vi "H5Diterate_cbhelper.vi"(5 "VI Refnum":refnum<vi>, 6 "error in (no error)":errorcluster, 7 "point":u64[](array[numeric]), 8 "User data in":variant, 9 "Data array in":variant) -> (0 "error out":errorcluster, 1 "Stop":i32(ring) items=["Error"=-1, "Continue"=0, "Stop"=1], 2 "User data out":variant, 3 "Data array out":variant)   [LabVIEW 2017]
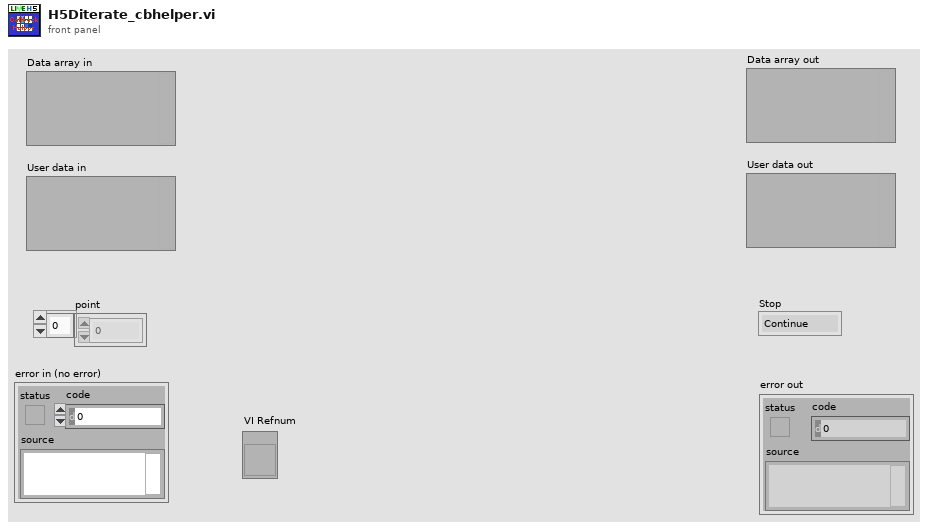
[diagram p1: front panel]
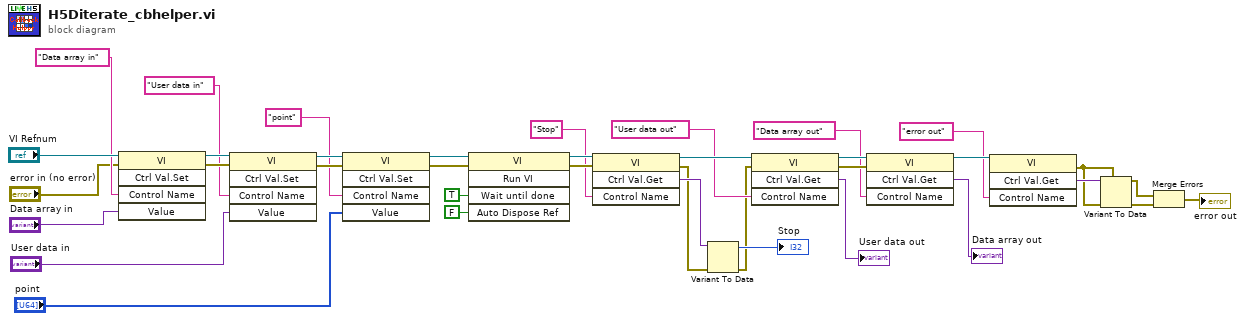
[diagram p0: block diagram]
diagram:
  n1 = invoke class="VI" method="Ctrl Val.Set"(reference="VI Refnum", error in="error in (no error)", "Control Name"="Data array in", "Value"="Data array in") -> (reference out=w34:refnum<vi>, error out=w33:errorcluster)  [unwired: 1 in, 3 out]
  n2 = invoke class="VI" method="Ctrl Val.Set"(reference=w34, error in=w33, "Control Name"="User data in", "Value"="User data in") -> (reference out=w30:refnum<vi>, error out=w29:errorcluster)  [unwired: 1 in, 3 out]
  n3 = invoke class="VI" method="Ctrl Val.Set"(reference=w30, error in=w29, "Control Name"="point", "Value"="point") -> (reference out=w25:refnum<vi>, error out=w24:errorcluster)  [unwired: 1 in, 3 out]
  n4 = invoke class="VI" method="Run VI"(reference=w25, error in=w24, "Wait until done"=TRUE ("Wait Until Done"), "Auto Dispose Ref"=FALSE ("Auto Dispose Reference")) -> (reference out=w21:refnum<vi>, error out=w20:errorcluster)  [unwired: 1 in, 3 out]
  n5 = invoke class="VI" method="Ctrl Val.Get"(reference=w21, error in=w20, "Control Name"="Stop") -> (reference out=w15:refnum<vi>, error out=w16:errorcluster, "Get Control Value Variant"=w18:variant)  [unwired: 1 in, 1 out]
  n6 = Variant To Data(error in=w16, Variant=w18) -> (data=→"Stop":i32, error out=w13:errorcluster)  [unwired: 1 in]
  n7 = invoke class="VI" method="Ctrl Val.Get"(reference=w15, error in=w13, "Control Name"="User data out") -> (reference out=w12:refnum<vi>, error out=w11:errorcluster, "Get Control Value Variant"=→"User data out":variant)  [unwired: 1 in, 1 out]
  n8 = invoke class="VI" method="Ctrl Val.Get"(reference=w12, error in=w11, "Control Name"="Data array out") -> (reference out=w7:refnum<vi>, "Get Control Value Variant"=→"Data array out":variant)  [unwired: 1 in, 2 out]
  n9 = invoke class="VI" method="Ctrl Val.Get"(reference=w7, "Control Name"="error out") -> (error out=w2:errorcluster, "Get Control Value Variant"=w5:variant)  [unwired: 2 in, 2 out]
  n10 = Variant To Data(error in=w2, type=w2, Variant=w5) -> (data=w3:errorcluster, error out=w4:errorcluster)
  n11 = Merge Errors(w3, w4) -> (→"error out":errorcluster)
